vi "Visa find resource.vi"() -> ()   [LabVIEW 2018]
panel:
  out "return count":u32
  out "find list":string[](array[string])
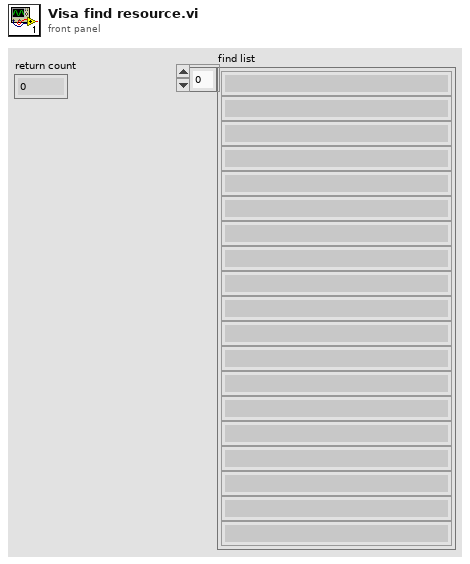
[diagram p1: front panel]
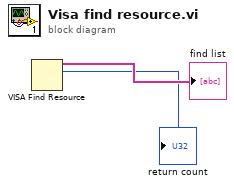
[diagram p0: block diagram]
diagram:
  n1 = VISA Find Resource() -> (2:→"return count":u32, 3:→"find list":string[])  [unwired: 3 in, 1 out]
